vi "ws_configure template keys.vi"() -> (2 "Template Keys":T1)   [LabVIEW 2011]
uses:
  Addons/internet/utils/keyedarr.llb/Keyed Array.ctl
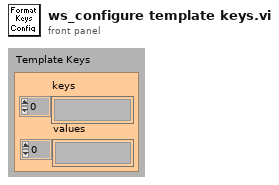
[diagram p1: front panel]
types:
  T1 = typedef "Keyed Array.ctl" = cluster{"keys":string[], "values":string[]}
  T2 = cluster{"key name":string, "key value":string, "default value":string}[]
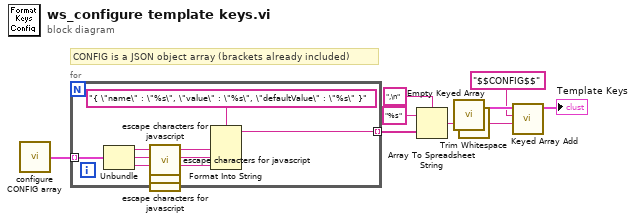
[diagram p0: block diagram]
diagram:
  # "CONFIG is a JSON object array (brackets already included)"
  n1 = call "configure CONFIG array.vi"() -> ("CONFIG"=w1:T2)
  n2 = for {
    tunnel: [w17] -> w7 mode=indexing
    tunnel: w1 -> [w16] mode=indexing
    n3 = Unbundle(w16) -> ("key name"=w15:string, "key value"=w13:string, "default value"=w11:string)
    n4 = call "escape characters for javascript.vi"("String (\"\")"=w15) -> ("escaped String"=w14:string)  [unwired: 4 in]
    n5 = call "escape characters for javascript.vi"("String (\"\")"=w13) -> ("escaped String"=w12:string)  [unwired: 4 in]
    n6 = call "escape characters for javascript.vi"("String (\"\")"=w11) -> ("escaped String"=w10:string)  [unwired: 4 in]
    n7 = Format Into String(format string="{ \"name\" : \"%s\", \"value\" : \"%s\", \"defaultValue\" : \"%s\" }", w14, w12, w10) -> (resulting string=w17:string)  [unwired: 2 in, 1 out]
  }
  n8 = Array To Spreadsheet String(delimiter (Tab)=",\n", array=w7, 3:"%s" ("format string")) -> (spreadsheet string=w4:string)
  n9 = call "Empty Keyed Array.vi"() -> ("empty keyed array"=w9:T1)  [unwired: 3 out]
  n10 = call <vilib>:"Trim Whitespace.vi"("string"=w4) -> ("trimmed string"=w3:string)  [unwired: 1 in]
  n11 = call "Keyed Array Add.vi"("value"=w3, "key"="$$CONFIG$$", "array in"=w9) -> ("array out"=→"Template Keys":T1)  [unwired: 1 in, 3 out]
